vi "Write Location.vi"(8 "error in (no error)":errorcluster, 10 "Location":i32[](array[numeric]), 11 "Array Location Mailman in":refnum<class "Array Location Mailman.lvclass">) -> (0 "error out":errorcluster, 3 "Array Location Mailman out":refnum<class "Array Location Mailman.lvclass">)   [LabVIEW 2019, in "Array Location Mailman.lvclass"]
uses:
  Array Location Mailman.lvclass
  Array Location Mailman.lvclass/Array Location Mailman.ctl
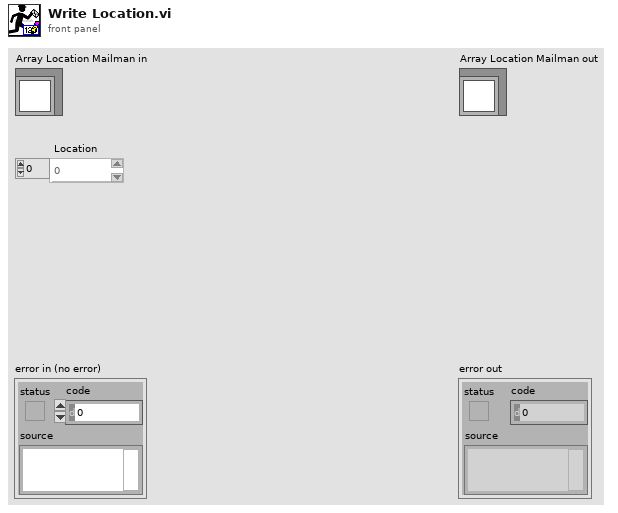
[diagram p1: front panel]
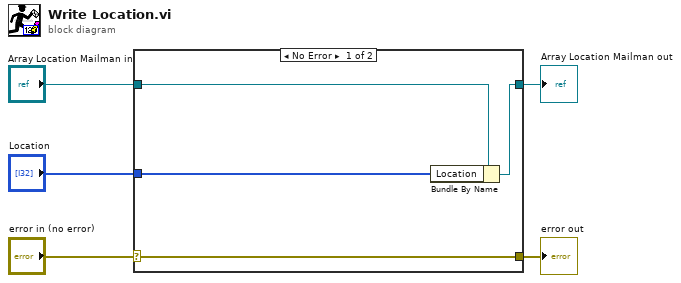
[diagram p0: block diagram]
diagram:
  n1 = case shown="No Error" "error in (no error)" {
    selector: "error in (no error)" -> [w9 w10]
    tunnel: [w9 w10] -> w4
    tunnel: [w7 w11] -> w2
    tunnel: "Array Location Mailman in" -> [w8 w11]
    tunnel: "Location" -> [w6 _]
    frame No Error {
      n2 = Bundle By Name(cluster=w8, "Location"=w6) -> (w7:refnum<class "Array Location Mailman.lvclass">)
    }
    frame Error {
    }
  }
  "error out" <- w4
  "Array Location Mailman out" <- w2
